vi "UART Read and Check Length.vi"(4 "Len":u8, 5 "error in (no error)":errorcluster, 6 "TimeOut(s)":dbl=3.0, 7 "ExpectStr":string="OK", 8 "VISA Resource In":refnum<visa-resource-name>="COM1") -> (0 "error out":errorcluster, 1 "OK?":bool, 2 "StrOut":string, 3 "VISA Resource Out":refnum<visa-resource-name>)   [LabVIEW 2015]
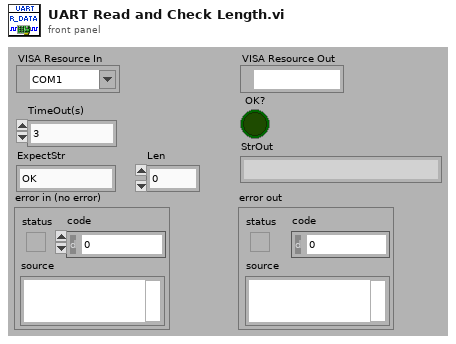
[diagram p1: front panel]
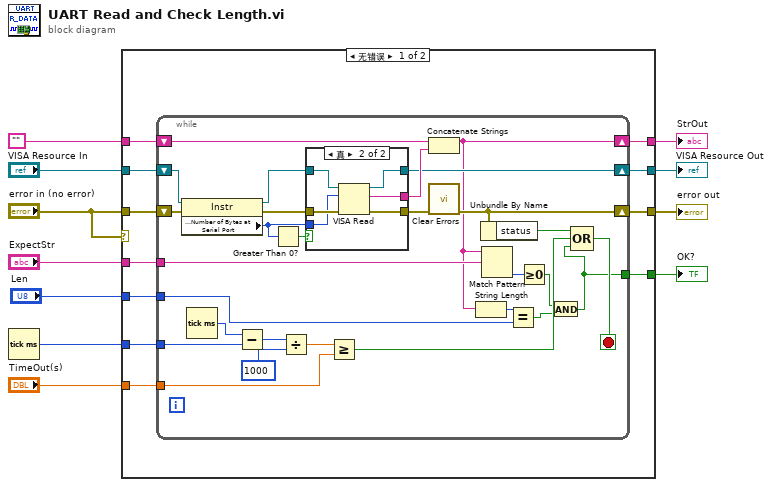
[diagram p0: block diagram]
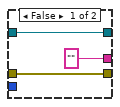
[diagram p2: hidden frame]
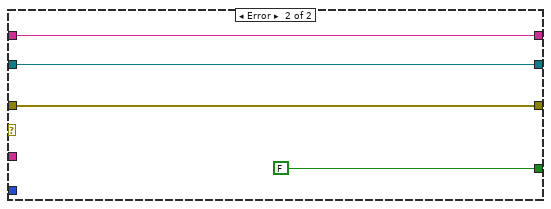
[diagram p3: hidden frame]
diagram:
  n1 = Tick Count (ms)() -> (millisecond timer value=w10:u32)
  n2 = case shown="无错误" "error in (no error)" {
    tunnel: "" -> [w22 w60]
    tunnel: w10 -> [w21 _]
    tunnel: "VISA Resource In" -> [w20 w63]
    tunnel: "error in (no error)" -> [w19 w62]
    tunnel: "ExpectStr" -> [w18 _]
    tunnel: [w17 w60] -> w7
    tunnel: [w16 w62] -> w6
    tunnel: [w15 w63] -> w5
    tunnel: "TimeOut(s)" -> [w14 _]
    tunnel: [w13 FALSE] -> w3
    tunnel: "Len" -> [w12 _]
    frame No Error {
      n3 = while {
        shift-right: [w29] -> w16
        shift-left: w19 -> [w48]
        shift-right: [w28] -> w17
        shift-left: w22 -> [w45]
        tunnel: w21 -> [w42]
        tunnel: w14 -> [w31]
        tunnel: w18 -> [w33]
        shift-right: [w32] -> w15
        shift-left: w20 -> [w36]
        tunnel: [w23] -> w13
        tunnel: w12 -> [w26]
        stop <- w37 stop-if-true
        n4 = property class="Instr"(reference=w36, error in=w48) -> (reference out=w49:refnum<visa-resource-name>, error out=w47:errorcluster, "Serial Settings:Number of Bytes at Serial Port"=w46:u32)
        n5 = Tick Count (ms)() -> (millisecond timer value=w43:u32)
        n6 = Subtract(x=w43, y=w42) -> (x-y=w34:u32)
        n7 = Greater Than 0?(x=w46) -> (x > 0?=w50:bool)
        n8 = Divide(x=w34, y=u32 1000) -> (x/y=w41:dbl)
        n9 = case shown="真" w50 {
          tunnel: w49 -> [w51 w59]
          tunnel: w47 -> [w53 w58]
          tunnel: w46 -> [_ w57]
          tunnel: [w53 w56] -> w40
          tunnel: [w51 w55] -> w32
          tunnel: ["" ("read buffer") w54] -> w44
          frame False {
          }
          frame True {
            n10 = VISA Read(VISA resource name=w59, byte count=w57, error in (no error)=w58) -> (VISA resource name out=w55:refnum<visa-resource-name>, read buffer=w54:string, error out=w56:errorcluster)  [unwired: 1 out]
          }
        }
        n11 = Greater Or Equal?(x=w41, y=w31) -> (x >= y?=w30:bool)
        n12 = Concatenate Strings(w45, w44) -> (w28:string)
        n13 = call <vilib>:"Clear Errors.vi"("error in (no error)"=w40) -> ("error out"=w29:errorcluster)  [unwired: 5 in, 1 out]
        n14 = String Length(string=w28) -> (length=w27:i32)
        n15 = Unbundle By Name(w29) -> ("status"=w38:bool)
        n16 = Match Pattern(string=w28, regular expression=w33) -> (offset past match=w39:i32)  [unwired: 1 in, 3 out]
        n17 = Equal?(x=w27, y=w26) -> (x = y?=w25:bool)
        n18 = Greater Or Equal To 0?(x=w39) -> (x >= 0?=w24:bool)
        n19 = And(x=w24, y=w25) -> (x .and. y?=w23:bool)
        n20 = Compound Arithmetic op=OR(w38, w30, w23) -> (w37:bool)
      }
    }
    frame Error {
    }
  }
  "StrOut" <- w7
  "VISA Resource Out" <- w5
  "error out" <- w6
  "OK?" <- w3
